vi "1DTo2D.vi"(8 "error in (no error)":errorcluster, 11 "reshapeInfo":T1) -> (0 "error in (no error) 2":errorcluster, 3 "Array out":i16[][](array[numeric]))   [LabVIEW 2020]
uses:
  reshapeINfo_TypDef.ctl
  emptyArray_TYpDEf.ctl
  emptyArrayCamX_TypDef.ctl
  reshapeArrayCommand_TypDEf.ctl
panel:
  out "Array out 3":dbl[][](graph)
  out "Array out 2":i16[][](graph)
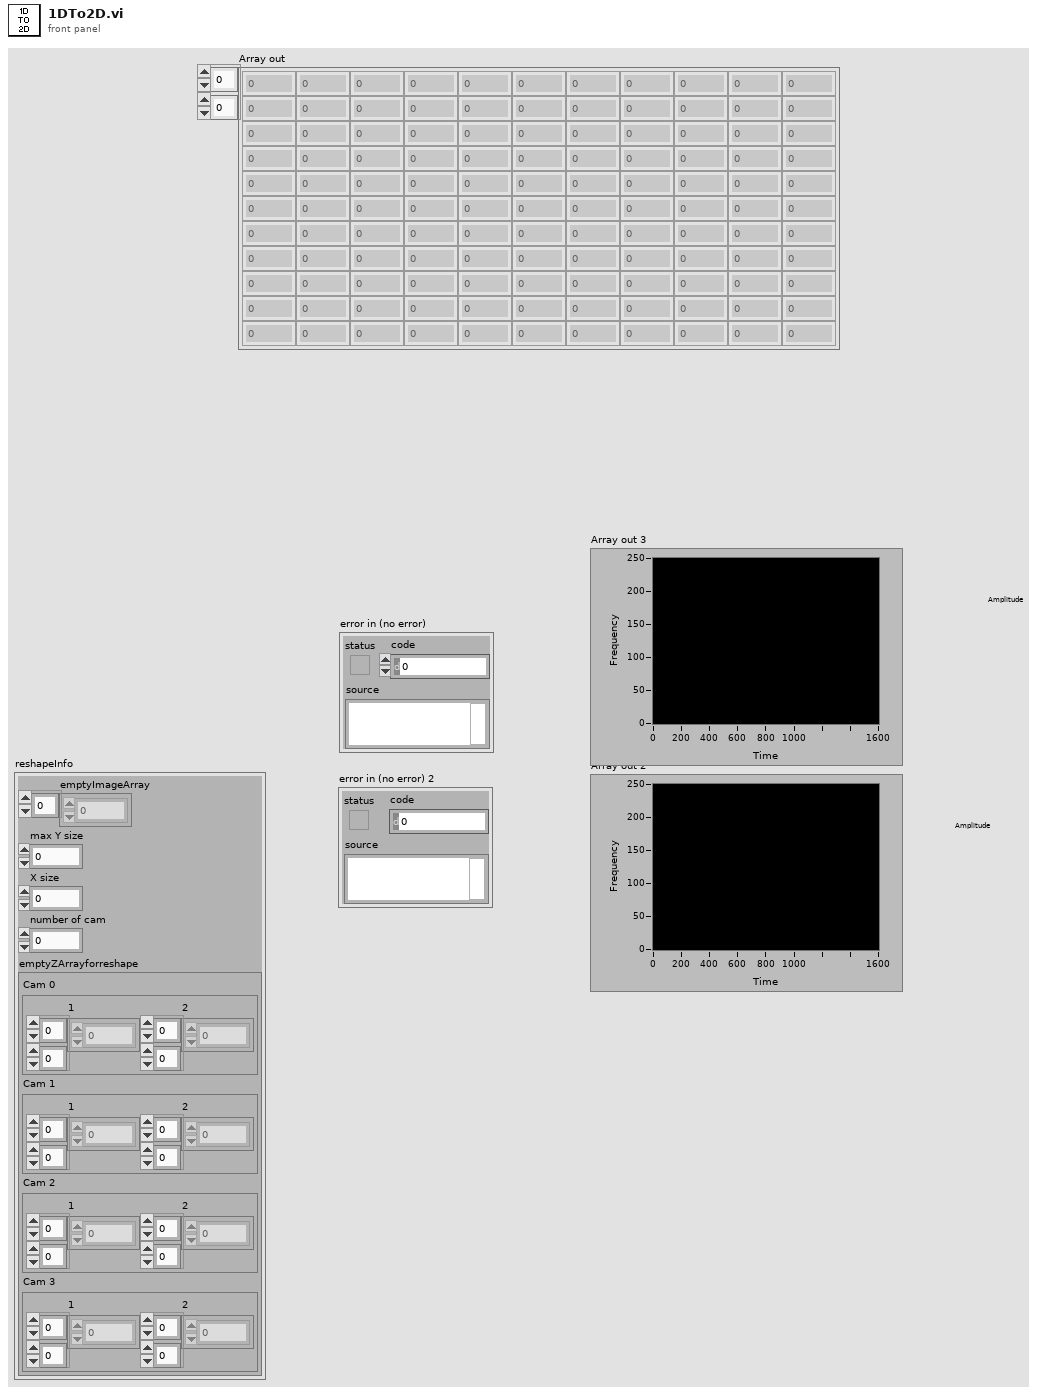
[diagram p1: front panel]
types:
  T1 = typedef "reshapeINfo_TypDef.ctl" = cluster{"emptyImageArray":dbl[], "max Y size":i32, "X size":i32, "number of cam":i32, "emptyZArrayforreshape":T2}
  T2 = typedef "emptyArray_TYpDEf.ctl" = cluster{"Cam 0":T3, "Cam 1":T3, "Cam 2":T3, "Cam 3":T3}
  T3 = typedef "emptyArrayCamX_TypDef.ctl" = cluster{"1":dbl[][], "2":dbl[][]}
  T4 = typedef "reshapeArrayCommand_TypDEf.ctl" = enum16{"init array", "addImage", "read", "init resolution"}
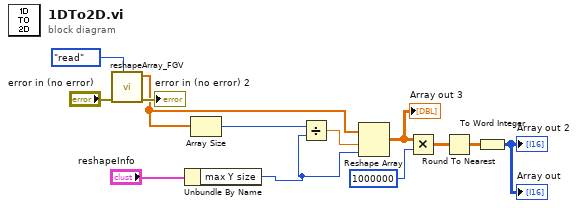
[diagram p0: block diagram]
diagram:
  n1 = call "reshapeArray_FGV.vi"("command"=reshapeArrayCommand_TypDEf."read", "error in (no error)"="error in (no error)") -> ("error in (no error) 2"=→"error in (no error) 2":errorcluster, "ImageArray"=w6:dbl[])  [unwired: 8 in]
  n2 = Unbundle By Name("reshapeInfo") -> ("max Y size"=w1:i32)
  n3 = Array Size(array=w6) -> (size(s)=w7:i32)
  n4 = Divide(x=w7, y=w1) -> (x/y=w5:dbl)
  n5 = Reshape Array(w6, w5, w1) -> (w2:dbl[][])
  "Array out 3" <- w2
  n6 = Multiply(x=w2, y=1000000 ("Numeric")) -> (x*y=w9:dbl[][])
  n7 = Round To Nearest(number=w9) -> (nearest integer value=w8:dbl[][])
  n8 = To Word Integer(number=w8) -> (16bit integer=→"Array out" →"Array out 2":i16[][])
